vi "In Range Limit.vi"(6 "Lower Limit":dbl, 7 "Upper Limit":dbl, 8 "Feedback":dbl, 9 "Motor In":dbl) -> (3 "Motor Out":dbl)   [LabVIEW 2011]
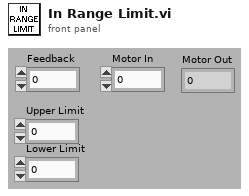
[diagram p1: front panel]
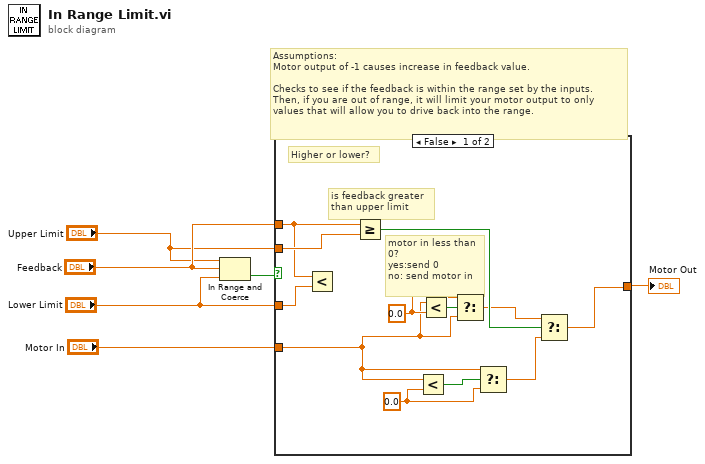
[diagram p0: block diagram]
diagram:
  # "Assumptions:\nMotor output of -1 causes increase in feedback value.\n\nChecks to see if the feedback is within the range set by the inputs.\nThen, if you are out of range, it will limit your motor output to only\nvalues that will allow you to drive back into the range."
  n1 = In Range and Coerce(upper limit="Upper Limit", x="Feedback", lower limit="Lower Limit") -> (In Range?=w4:bool)  [unwired: 1 out]
  n2 = case shown="False" w4 {
    tunnel: [w11 w19] -> w1
    tunnel: "Motor In" -> [w7 w19]
    tunnel: "Upper Limit" -> [w10 _]
    tunnel: "Feedback" -> [w9 _]
    tunnel: "Lower Limit" -> [w8 _]
    frame False {
      w13 = 0.0 ("y")
      w16 = 0.0 ("y")
      # "motor in less than\n0? \nyes:send 0\nno: send motor in"
      # "is feedback greater \nthan upper limit"
      # "Higher or lower?"
      n3 = Less?(x=w9, y=w8) -> ()  [unwired: 1 out]
      n4 = Greater Or Equal?(x=w9, y=w10) -> (x >= y?=w18:bool)
      n5 = Less?(x=w7, y=w13) -> (x < y?=w14:bool)
      n6 = Less?(x=w7, y=w16) -> (x < y?=w17:bool)
      n7 = Select(t=w16, s=w17, f=w7) -> (s? t:f=w15:dbl)
      n8 = Select(t=w7, s=w14, f=w13) -> (s? t:f=w12:dbl)
      n9 = Select(t=w15, s=w18, f=w12) -> (s? t:f=w11:dbl)
    }
    frame True {
    }
  }
  "Motor Out" <- w1
